vi "Timer.vi"(0 "Time_Required":i32, 11 "Error_In":errorcluster, 13 "Timer_Select":T1=enum."Time_Out?") -> (4 "Time_Out?":bool, 6 "Time":dbl, 8 "Start?":bool, 15 "Error_Out":errorcluster)   [LabVIEW 2023]
doc: "Used for timer opertion."
uses:
  Controls/Timer_Operation_Select.ctl
  Controls/Timer_Data.ctl
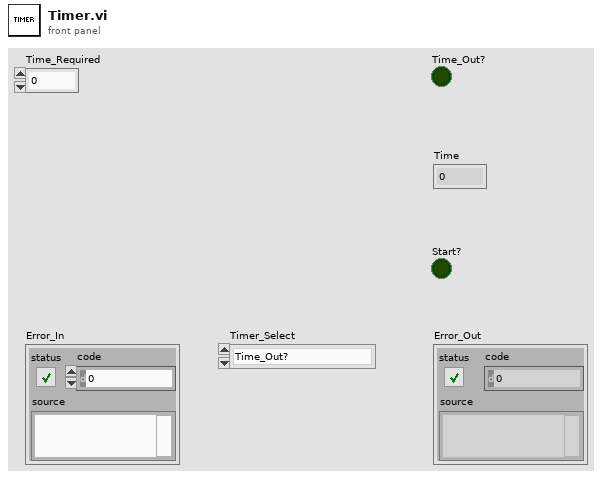
[diagram p1: front panel]
types:
  T1 = typedef "Timer_Operation_Select.ctl" = enum16{"Start_Timer", "Pause_Timer", "Time_Out?", "Stop_Timer"}
  T2 = typedef "Timer_Data.ctl" = cluster{"Start_Time":dbl, "Start?":bool, "Wait_Time":dbl, "Time":dbl}
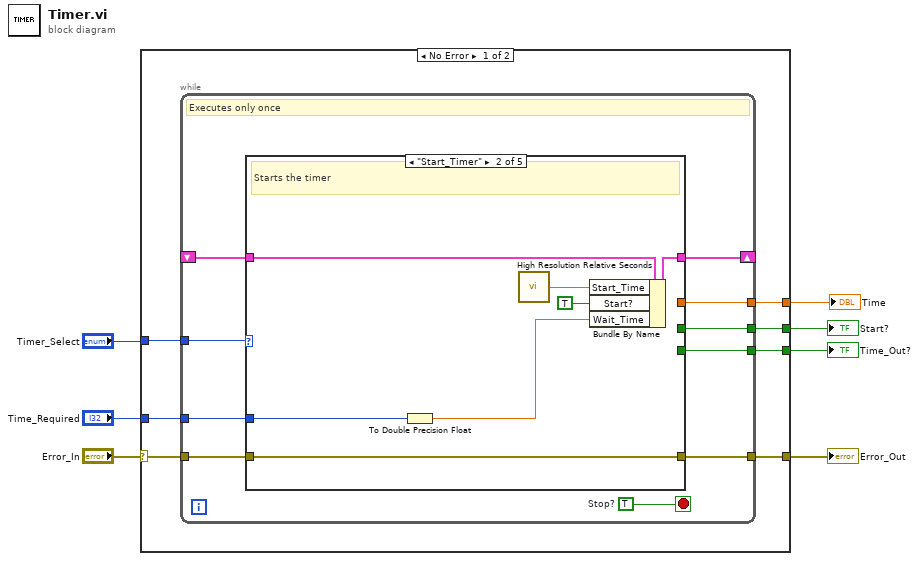
[diagram p0: block diagram]
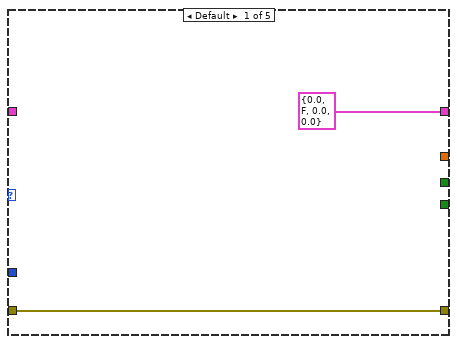
[diagram p2: hidden frame]
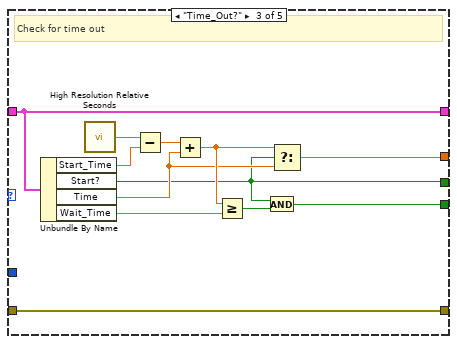
[diagram p3: hidden frame]
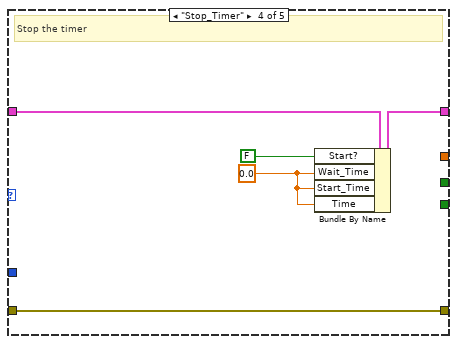
[diagram p4: hidden frame]
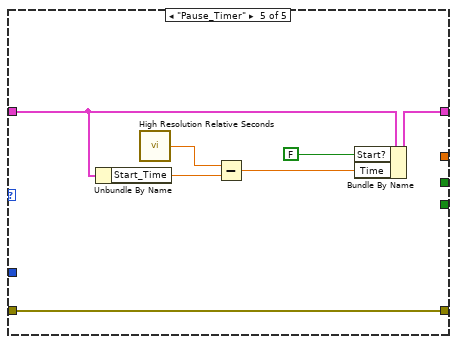
[diagram p5: hidden frame]
diagram:
  n1 = case shown="No Error" "Error_In" {
    selector: "Error_In" -> [w10 w58]
    tunnel: [w14 _] -> w2
    tunnel: [w13 w58] -> w6
    tunnel: "Time_Required" -> [w12 _]
    tunnel: "Timer_Select" -> [w11 _]
    tunnel: [w9 _] -> w3
    tunnel: [w8 _] -> w1
    frame No Error {
      n2 = while {
        tunnel: w11 -> [w24]
        shift-right: [w23] -> _
        shift-left: _ -> [w22]
        tunnel: [w21] -> w14
        tunnel: w10 -> [w19]
        tunnel: [w18] -> w13
        tunnel: w12 -> [w17]
        tunnel: [w16] -> w9
        tunnel: [w15] -> w8
        stop <- w20 stop-if-true
        w20 = TRUE  # Stop?
        # "Executes only once"
        n3 = case shown="\"Start_Timer\"" w24 {
          tunnel: [T2 {"Start_Time"=0.0, "Start?"=FALSE, "Wait_Time"=0.0, "Time"=0.0} ("Cluster") w31 w34 w48 w57] -> w23
          tunnel: w22 -> [_ w32 w34 w49 w54]
          tunnel: [_ _ w42 _ _] -> w21
          tunnel: w19 -> [w26 w33 w44 w50 w55]
          tunnel: [w26 w33 w44 w50 w55] -> w18
          tunnel: w17 -> [_ w28 _ _ _]
          tunnel: [_ _ w35 _ _] -> w16
          tunnel: [_ _ w36 _ _] -> w15
          frame Default {
          }
          frame "Start_Timer" {
            # "Starts the timer"
            n4 = To Double Precision Float(number=w28) -> (double precision float=w27:dbl)
            n5 = call <vilib>:"High Resolution Relative Seconds.vi"() -> ("relative seconds"=w30:dbl)
            n6 = Bundle By Name(cluster=w32, "Start_Time"=w30, "Start?"=TRUE, "Wait_Time"=w27) -> (w31:T2)
          }
          frame "Time_Out?" {
            # "Check for time out"
            n7 = Unbundle By Name(w34) -> ("Start_Time"=w40:dbl, "Start?"=w36:bool, "Time"=w37:dbl, "Wait_Time"=w38:dbl)
            n8 = call <vilib>:"High Resolution Relative Seconds.vi"() -> ("relative seconds"=w43:dbl)
            n9 = Subtract(x=w43, y=w40) -> (x-y=w41:dbl)
            n10 = Add(x=w41, y=w37) -> (x+y=w39:dbl)
            n11 = Greater Or Equal?(x=w39, y=w38) -> (x >= y?=w45:bool)
            n12 = And(x=w36, y=w45) -> (x .and. y?=w42:bool)
            n13 = Select(t=w39, s=w36, f=w37) -> (s? t:f=w35:dbl)
          }
          frame "Stop_Timer" {
            w46 = 0.0 ("Wait_Time")
            # "Stop the timer"
            n14 = Bundle By Name(cluster=w49, "Start?"=FALSE, "Wait_Time"=w46, "Start_Time"=w46, "Time"=w46) -> (w48:T2)
          }
          frame "Pause_Timer" {
            n15 = Unbundle By Name(w54) -> ("Start_Time"=w53:dbl)
            n16 = call <vilib>:"High Resolution Relative Seconds.vi"() -> ("relative seconds"=w52:dbl)
            n17 = Subtract(x=w52, y=w53) -> (x-y=w51:dbl)
            n18 = Bundle By Name(cluster=w54, "Start?"=FALSE, "Time"=w51) -> (w57:T2)
          }
        }
      }
    }
    frame Error {
    }
  }
  "Error_Out" <- w6
  "Time_Out?" <- w2
  "Time" <- w3
  "Start?" <- w1
